vi "Open.vi"(8 "error in (no error)":errorcluster caption="entrée d'erreur (pas d'erreur)", 11 "Class UART (Default) en entrée":refnum<class "Class UART (Default).lvclass">) -> (0 "error out":errorcluster caption="sortie d'erreur", 3 "Class UART (Default) en sortie":refnum<class "Class UART (Default).lvclass">)   [LabVIEW 2020, in "Library Instrument & Equipement.lvlib" / "Library UART.lvlib" / "Class UART (Default).lvclass"]
uses:
  Class UART (Default).lvclass
  Class UART (Default).lvclass/Class UART (Default).ctl
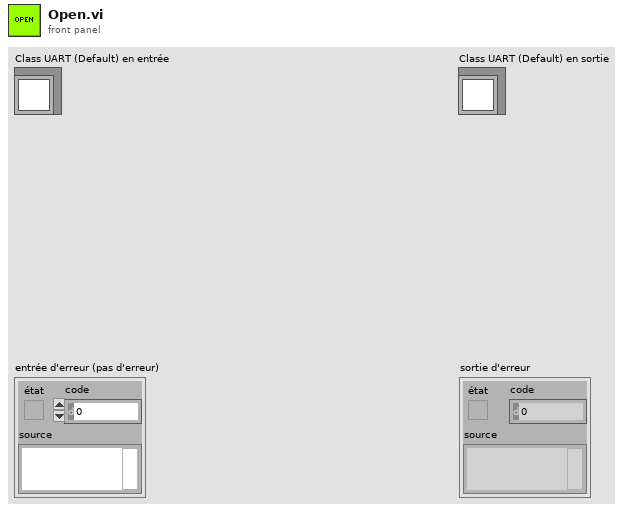
[diagram p1: front panel]
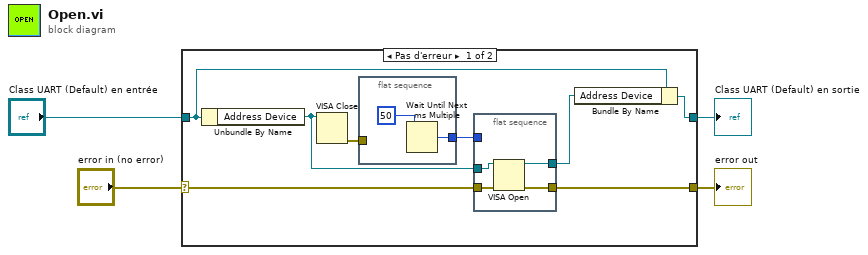
[diagram p0: block diagram]
diagram:
  n1 = case shown="Pas d'erreur" "error in (no error)" {
    selector: "error in (no error)" -> [w7 w20]
    tunnel: [w11 w20] -> w3
    tunnel: [w9 w19] -> w1
    tunnel: "Class UART (Default) en entrée" -> [w10 w19]
    frame No Error {
      n2 = Unbundle By Name(w10) -> ("Address Device"=w12:refnum<visa-resource-name>)
      n3 = VISA Close(VISA resource name=w12) -> (error out=w5:errorcluster)  [unwired: 1 in]
      n4 = flat-sequence {
        tunnel: [w14] -> w6
        tunnel: w5 -> [_]
        frame #0 {
          n5 = Wait Until Next ms Multiple(millisecond multiple=u32 50 ("milliseconds to wait")) -> (millisecond timer value=w14:u32)
        }
      }
      n6 = flat-sequence {
        tunnel: w12 -> [w18]
        tunnel: [w17] -> w11
        tunnel: [w16] -> w8
        tunnel: w7 -> [w15]
        tunnel: w6 -> [_]
        frame #0 {
          n7 = VISA Open(error in (no error)=w15, VISA resource name=w18) -> (VISA resource name=w16:refnum<visa-resource-name>, error out=w17:errorcluster)  [unwired: 3 in]
        }
      }
      n8 = Bundle By Name(cluster=w10, "Address Device"=w8) -> (w9:refnum<class "Class UART (Default).lvclass">)
    }
    frame Error {
    }
  }
  "error out" <- w3
  "Class UART (Default) en sortie" <- w1
